vi "Configure Measurement Characteristics (Eye Pattern).vi"(0 "VISA resource name":refnum<visa-resource-name>, 1 "Eye Window Stop (60%)":i32=60, 5 "Eye Window Start (40%)":i32=40, 7 "Start Measurement After (1 hit)":i32=1, 11 "error in (no error)":errorcluster, 12 "Waveform Source (0: Channel 1)":i32(ring) items=["Channel 1", "Channel 2", "Channel 3", "Channel 4", "Common 1", "Common 2", "Differential 1", "Differential 2", "Memory 1", "Memory 2", "Memory 3", "Memory 4", "Function 1", "Function 2", "Function 3", "Function 4", "Function 5", "Function 6", "Function 7", "Function 8", "Function 9", "Function 10", "Function 11", "Function 12", "Function 13", "Function 14", "Function 15", "Function 16", "Clock", "Equalized", "MTRend", "MSPectrum"]) -> (4 "VISA resource name out":refnum<visa-resource-name>, 15 "error out":errorcluster)   [LabVIEW 2020, in "Agilent 90000 Series.lvlib"]
doc: "Configure eye pattern definition for color grade math operation. It configures eye window start,eye window stop and eye window stop after properties."
uses:
  Agilent 90000 Series.lvlib
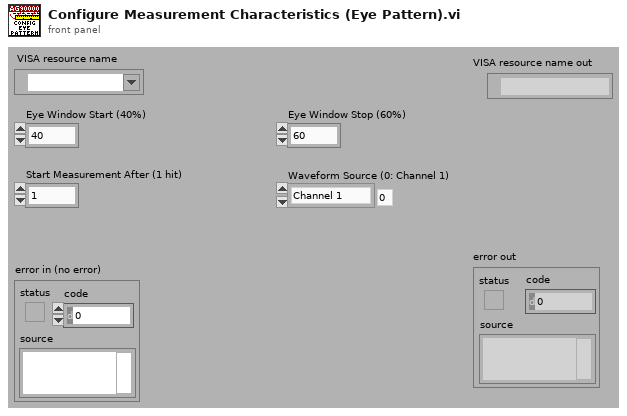
[diagram p1: front panel]
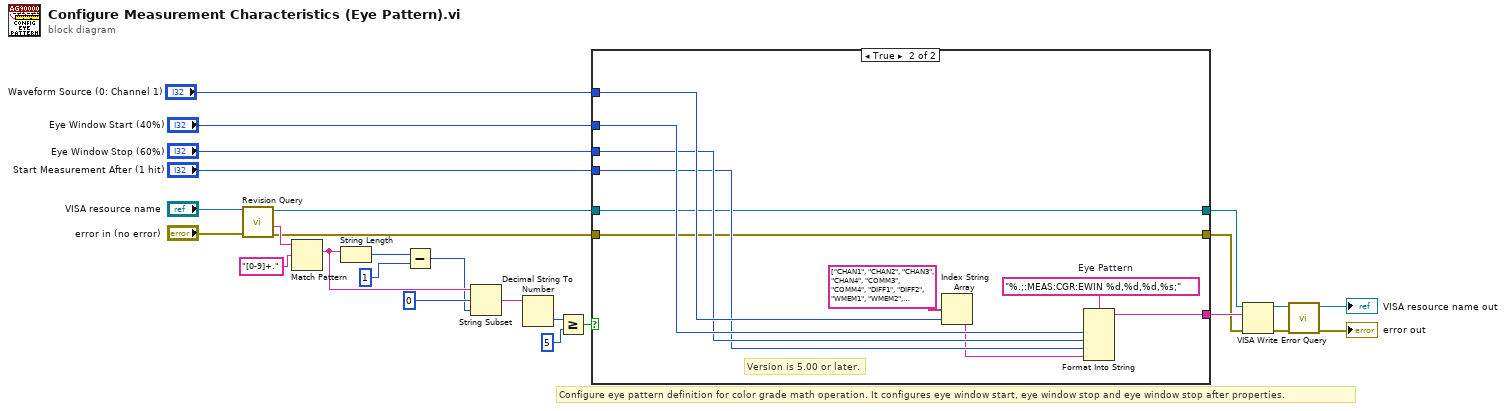
[diagram p0: block diagram]
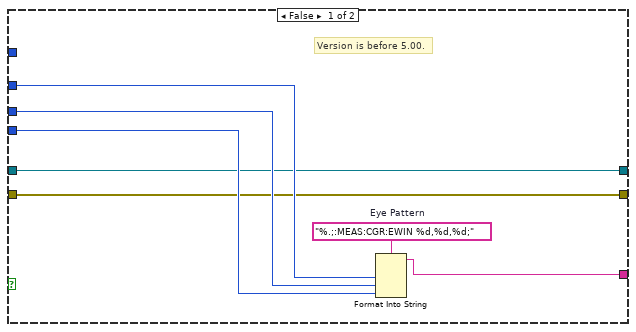
[diagram p2: hidden frame]
diagram:
  # "Configure eye pattern definition for color grade math operation. It configures eye window start, eye window stop and eye window stop after properties."
  n1 = call "Revision Query.vi"("error in (no error)"="error in (no error)", "VISA resource name"="VISA resource name") -> ("error out"=w4:errorcluster, "Instrument Firmware Revision"=w13:string, "VISA resource name out"=w6:refnum<visa-resource-name>)  [unwired: 6 in, 1 out]
  n2 = Match Pattern(string=w13, regular expression="[0-9]+.") -> (match substring=w21:string)  [unwired: 1 in, 3 out]
  n3 = String Length(string=w21) -> (length=w19:i32)
  n4 = Subtract(x=w19, y=1) -> (x-y=w17:i32)
  n5 = String Subset(string=w21, offset (0)=0, length (rest)=w17) -> (substring=w16:string)
  n6 = Decimal String To Number(string=w16) -> (number=w15:i32)  [unwired: 2 in, 1 out]
  n7 = Greater Or Equal?(x=w15, y=5) -> (x >= y?=w1:bool)
  n8 = case shown="True" w1 {
    tunnel: "Eye Window Start (40%)" -> [w32 w40]
    tunnel: "Eye Window Stop (60%)" -> [w31 w39]
    tunnel: "Start Measurement After (1 hit)" -> [w30 w38]
    tunnel: [w27 w36] -> w7
    tunnel: w6 -> [w29 w35]
    tunnel: [w29 w35] -> w5
    tunnel: w4 -> [w28 w34]
    tunnel: [w28 w34] -> w3
    tunnel: "Waveform Source (0: Channel 1)" -> [_ w42]
    frame False {
      w33 = "%.;:MEAS:CGR:EWIN %d,%d,%d;"  # Eye Pattern
      # "Version is before 5.00."
      n9 = Format Into String(format string=w33, w32, w31, w30) -> (resulting string=w27:string)  [unwired: 2 in, 1 out]
    }
    frame True {
      w43 = "%.;:MEAS:CGR:EWIN %d,%d,%d,%s;"  # Eye Pattern
      # "Version is 5.00 or later."
      n10 = Index String Array(1:w42, 2:string[] ["CHAN1", "CHAN2", "CHAN3", "CHAN4", "COMM3", "COMM4", "DIFF1", "DIFF2", "WMEM1", "WMEM2", "WMEM3", "WMEM4", "FUNC1", "FUNC2", "FUNC3", "FUNC4", "FUNC5", "FUNC6", "FUNC7", "FUNC8", "FUNC9", "FUNC10", "FUNC11", "FUNC12", "FUNC13", "FUNC14", "FUNC15", "FUNC16", "CLOC", "EQU", "MTR", "MSP"] ("string array")) -> (0:w37:string)  [unwired: 1 in]
      n11 = Format Into String(format string=w43, w40, w39, w38, w37) -> (resulting string=w36:string)  [unwired: 2 in, 1 out]
    }
  }
  n12 = VISA Write(VISA resource name=w5, write buffer=w7, error in (no error)=w3) -> (VISA resource name out=w24:refnum<visa-resource-name>, error out=w23:errorcluster)  [unwired: 1 out]
  n13 = call "Error Query.vi"("error in (no error)"=w23, "VISA resource name"=w24) -> ("error out"=→"error out":errorcluster, "VISA resource name out"=→"VISA resource name out":refnum<visa-resource-name>)  [unwired: 8 out]
